vi "Get All Frame and Signal Names.vi"(0 "XNET Cluster":refnum<k21>, 11 "error in":errorcluster) -> (3 "Cluster":string, 4 "Frame Names":string[](array[string]), 6 "Number of Frames":i32, 8 "Signal Names":string[][](array[string]), 10 "Number of Signals":i32[](array[numeric]), 15 "error out":errorcluster)   [LabVIEW 2018, in "Library-Ctrl.lvlib"]
uses:
  Library-Ctrl.lvlib
  <resource>/objmgr/xnet.rc
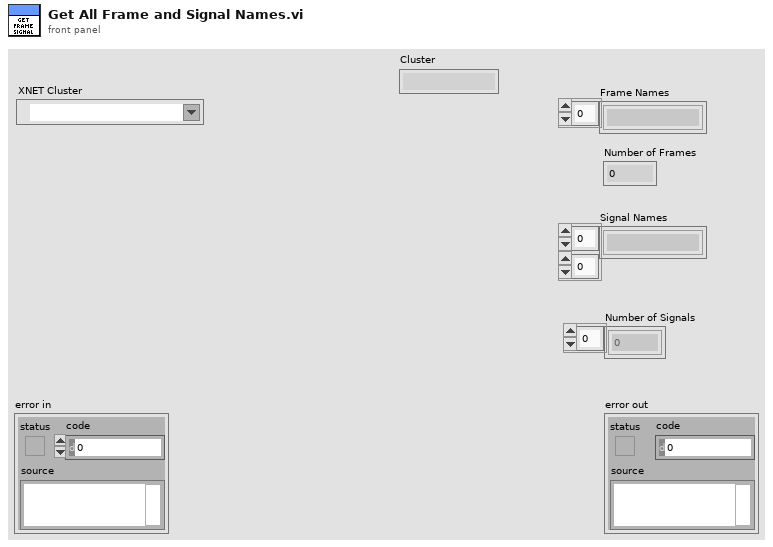
[diagram p1: front panel]
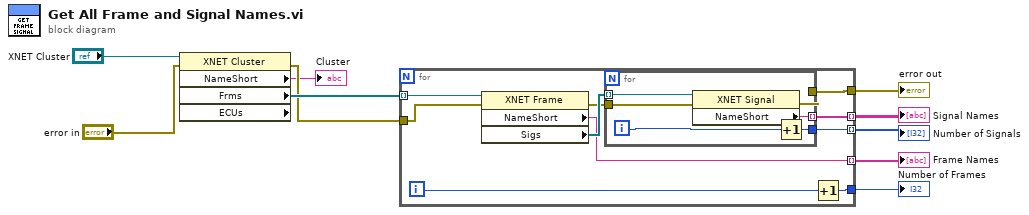
[diagram p0: block diagram]
diagram:
  n1 = property class="XNET Cluster" props=["NameShort", "Frms", "ECUs"](reference="XNET Cluster", error in="error in") -> (error out=w2:errorcluster, "NameShort"=→"Cluster":string, "Frms"=w4:refnum<k21>[])  [unwired: 2 out]
  n2 = for {
    tunnel: w4 -> [w12] mode=indexing
    tunnel: [w19] -> w8
    tunnel: w2 -> [w11]
    tunnel: [w17] -> w9 mode=indexing
    tunnel: [w16] -> w10 mode=indexing
    tunnel: [w15] -> w7 mode=indexing
    tunnel: [w14] -> w6
    i -> [w13]
    n3 = property class="XNET Frame"(reference=w12, error in=w11) -> (error out=w18:errorcluster, "NameShort"=w16:string, "Sigs"=w20:refnum<k21>[])  [unwired: 1 out]
    n4 = for {
      tunnel: w20 -> [w22] mode=indexing
      tunnel: [w26] -> w19
      tunnel: w18 -> [w21]
      tunnel: [w25] -> w17 mode=indexing
      tunnel: [w23] -> w15
      i -> [w24]
      n5 = property class="XNET Signal"(reference=w22, error in=w21) -> (error out=w26:errorcluster, "NameShort"=w25:string)  [unwired: 1 out]
      n6 = Increment(x=w24) -> (x+1=w23:i32)
    }
    n7 = Increment(x=w13) -> (x+1=w14:i32)
  }
  "Frame Names" <- w10
  "Signal Names" <- w9
  "error out" <- w8
  "Number of Frames" <- w6
  "Number of Signals" <- w7
